vi "Sound_Read_from_File.vi"() -> ()   [LabVIEW 2020]
panel:
  out "Sound Waveform - Channel 2":waveform(dbl)(graph)
  out "Sound Waveform - Channel 1":waveform(dbl)(graph)
  out "WAV file path":path
  out "Samples Read":i32
  # "Read Sound Data"
  # "Auther: Suparat Yeamkuan\nOverview: Read sound data (WAV file).\nRequirements: -"
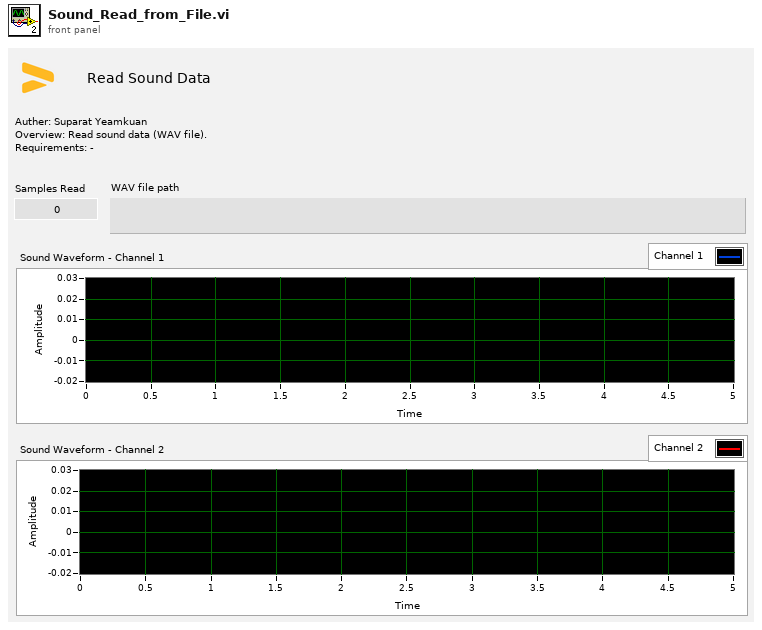
[diagram p1: front panel]
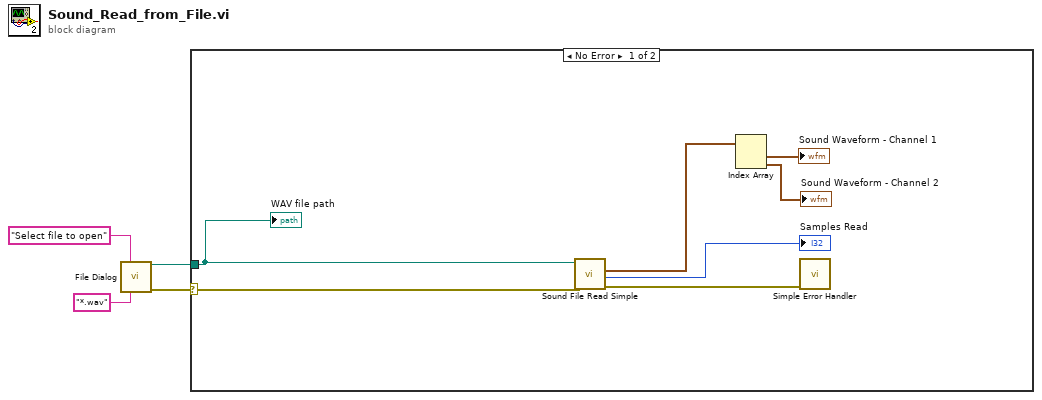
[diagram p0: block diagram]
diagram:
  n1 = call "File Dialog"("prompt"="Select file to open", "pattern (all files)"="*.wav") -> ("selected path"=w2:path, "error out"=w1:errorcluster)  [unwired: 10 in, 2 out]
  n2 = case shown="No Error" w1 {
    selector: w1 -> [w5 _]
    tunnel: w2 -> [w6 _]
    frame No Error {
      n3 = call <vilib>:"Sound File Read Simple.vi"("error in (no error)"=w5, "path"=w6) -> ("error out"=w10:errorcluster, "offset"=→"Samples Read":i32, "data"=w7:waveform(dbl)[])  [unwired: 6 in, 1 out]
      n4 = Index Array(array=w7) -> (element #1=→"Sound Waveform - Channel 1":waveform(dbl), element #2=→"Sound Waveform - Channel 2":waveform(dbl))  [unwired: 2 in]
      n5 = call <vilib>:"Simple Error Handler.vi"("error in (no error)"=w10) -> ()  [unwired: 4 in, 5 out]
      "WAV file path" <- w6
    }
    frame Error {
    }
  }
